vi "Shift data Read.vi"(11 "input cluster":T2) -> (2 "output cluster":T1)   [LabVIEW 2015]
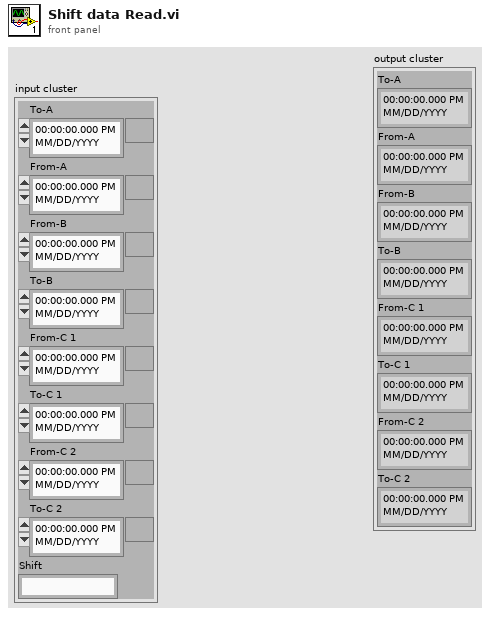
[diagram p1: front panel]
types:
  T1 = cluster{"To-A":timestamp, "From-A":timestamp, "From-B":timestamp, "To-B":timestamp, "From-C 1":timestamp, "To-C 1":timestamp, "From-C 2":timestamp, "To-C 2":timestamp}
  T2 = cluster{"To-A":timestamp, "From-A":timestamp, "From-B":timestamp, "To-B":timestamp, "From-C 1":timestamp, "To-C 1":timestamp, "From-C 2":timestamp, "To-C 2":timestamp, "Shift":string}
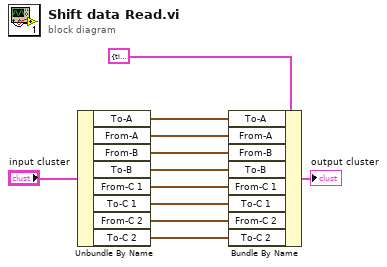
[diagram p0: block diagram]
diagram:
  n1 = Unbundle By Name("input cluster") -> ("To-A"=w3:timestamp, "From-A"=w4:timestamp, "From-B"=w5:timestamp, "To-B"=w6:timestamp, "From-C 1"=w7:timestamp, "To-C 1"=w8:timestamp, "From-C 2"=w10:timestamp, "To-C 2"=w9:timestamp)
  n2 = Bundle By Name(cluster=T1 {"To-A"=timestamp(0 s since 1904-01-01), "From-A"=timestamp(0 s since 1904-01-01), "From-B"=timestamp(0 s since 1904-01-01), "To-B"=timestamp(0 s since 1904-01-01), "From-C 1"=timestamp(0 s since 1904-01-01), "To-C 1"=timestamp(0 s since 1904-01-01), "From-C 2"=timestamp(0 s since 1904-01-01), "To-C 2"=timestamp(0 s since 1904-01-01)} ("input cluster"), "To-A"=w3, "From-A"=w4, "From-B"=w5, "To-B"=w6, "From-C 1"=w7, "To-C 1"=w8, "From-C 2"=w10, "To-C 2"=w9) -> (→"output cluster":T1)
